vi "Run.vi"(8 "error in (no error)":errorcluster, 10 "OTP Cluster Out":T1, 11 "RF Powers in":refnum<class "RF Power.lvclass">) -> (0 "error out":errorcluster, 1 "Parameters":cluster{"Name":string, "Value":string}[](array[cluster]), 2 "Canceled":bool, 3 "RF Powers out":refnum<class "RF Power.lvclass">)   [LabVIEW 2020, in "RF Power.lvclass"]
doc: "This is the main test vi. It is here that the test is implemented."
uses:
  RF Power.lvclass
  Measurement.lvclass
  Devices/Device.lvclass
  Devices/Controls/Change setting mode enum.ctl
  Devices/PIC-device/PIC-Device.lvclass
  Support VI/Update parameters (single).vi
  Instruments/Power Supply/Power Supply.lvclass
  Support VI/Update parameters (array).vi
  Instruments/Digital Multimeter/Digital Multimeter.lvclass
  XML Handler/XML Handler.lvclass
  Path Control/Paths.ctl
  Path Control/PathControl.lvclass
  Instruments/Signal Generator/Signal Generator.lvclass
  Controls/Loop order.ctl
  Controls/Run states.ctl
  Instruments/Power Meter/Power Meter.lvclass
  C:/Sandbox/Git_Sandbox/WiSpry Test Framework source code (LV20)/WiSpry Test Framework/Measurements/Measurement.lvclass
  Controls/OTP_Cluster.ctl
panel:
  in  "Cancel Button":bool
  out "Power Meter reading (dBm)":dbl[](array[numeric])
  out "Estimated finish time":timestamp format="%<%X>T"
  out "Parameters":string
  out "Current Frequency [Hz]":dbl format="%#_6p"
  out "Current Power [dBm]":dbl
  out "XY Graph":cluster{dbl[], dbl[]}[](graph)
  out "Progress":u8(slide) scale=0.0..100.0
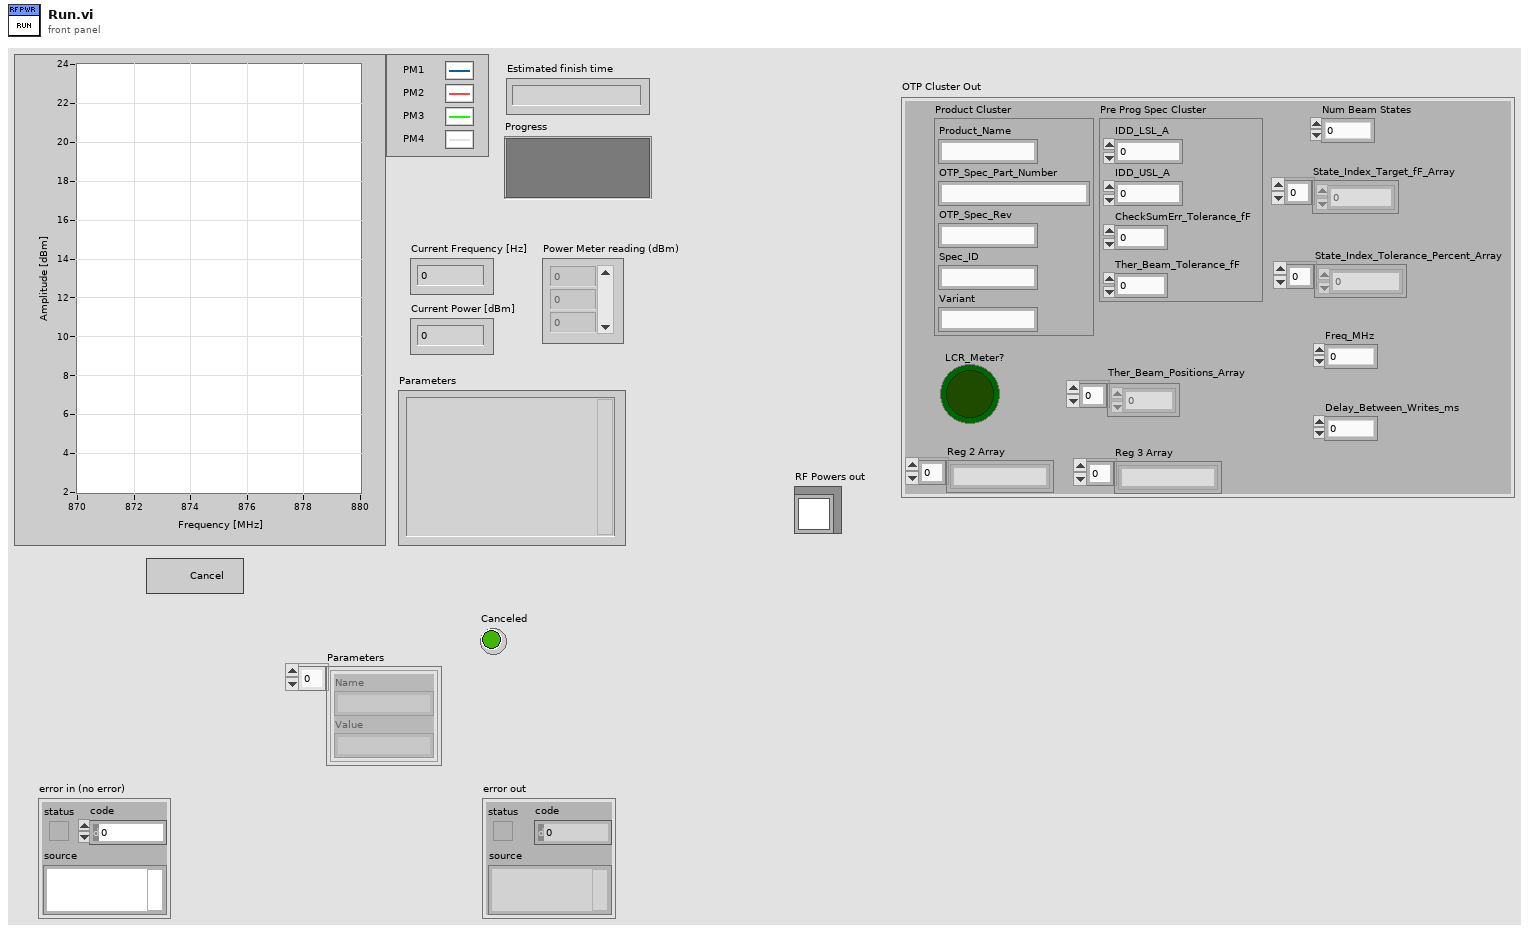
[diagram p1: front panel]
types:
  T1 = typedef "OTP_Cluster.ctl" = cluster{"Product Cluster":cluster{"Product_Name":string, "OTP_Spec_Part_Number":string, "OTP_Spec_Rev":string, "Spec_ID":string, "Variant":string}, "Pre Prog Spec Cluster":cluster{"IDD_LSL_A":dbl, "IDD_USL_A":dbl, "CheckSumErr_Tolerance_fF":dbl, "Ther_Beam_Tolerance_fF":dbl}, "LCR_Meter?":bool, "Reg 2 Array":string[], "Reg 3 Array":string[], "Num Beam States":i32, "State_Index_Target_fF_Array":dbl[], "State_Index_Tolerance_Percent_Array":dbl[], "Freq_MHz":dbl, "Delay_Between_Writes_ms":i32, "Ther_Beam_Positions_Array":i8[]}
  T2 = typedef "RF Power.lvclass/Run states.ctl" = enum16{"Init", "Set Device", "Set Power", "Set Frequency", "Read Environment", "Measure", "Done"}
  T3 = typedef "RF Power.lvclass/Loop order.ctl" = enum16{"Device -> Power -> Frequency", "Device -> Frequency -> Power"}
  T4 = enum32{"Invalid", "Standard", "Closed", "Hidden", "Minimized", "Maximized"}
  T5 = typedef "PIC-Device.lvclass/Change setting mode enum.ctl" = enum16{"Init", "Next", "Reset"}
  T6 = typedef "PathControl.lvclass/Paths.ctl" = enum16{"SigGen 1 -> DUT", "SigGen 2 -> DUT", "SigGen 1 -> PM 1", "SigGen 1 -> PM 2", "DUT -> SA", "DUT -> PM 2", "VSG -> DUT", "SigGen 2 -> PM 1", "SigGen 2 -> PM 2"}
  T7 = typedef "RF Power.lvclass/Config info.ctl" = cluster{"Frequency (MHz)":string, "Power (dBm)":string, "Loop order":T3, "SG loss":bool, "PM loss":bool, "SG":i32}
  T8 = typedef "XML Handler.lvclass/Result Cluster.ctl" = cluster{"Name":string, "Value":string}
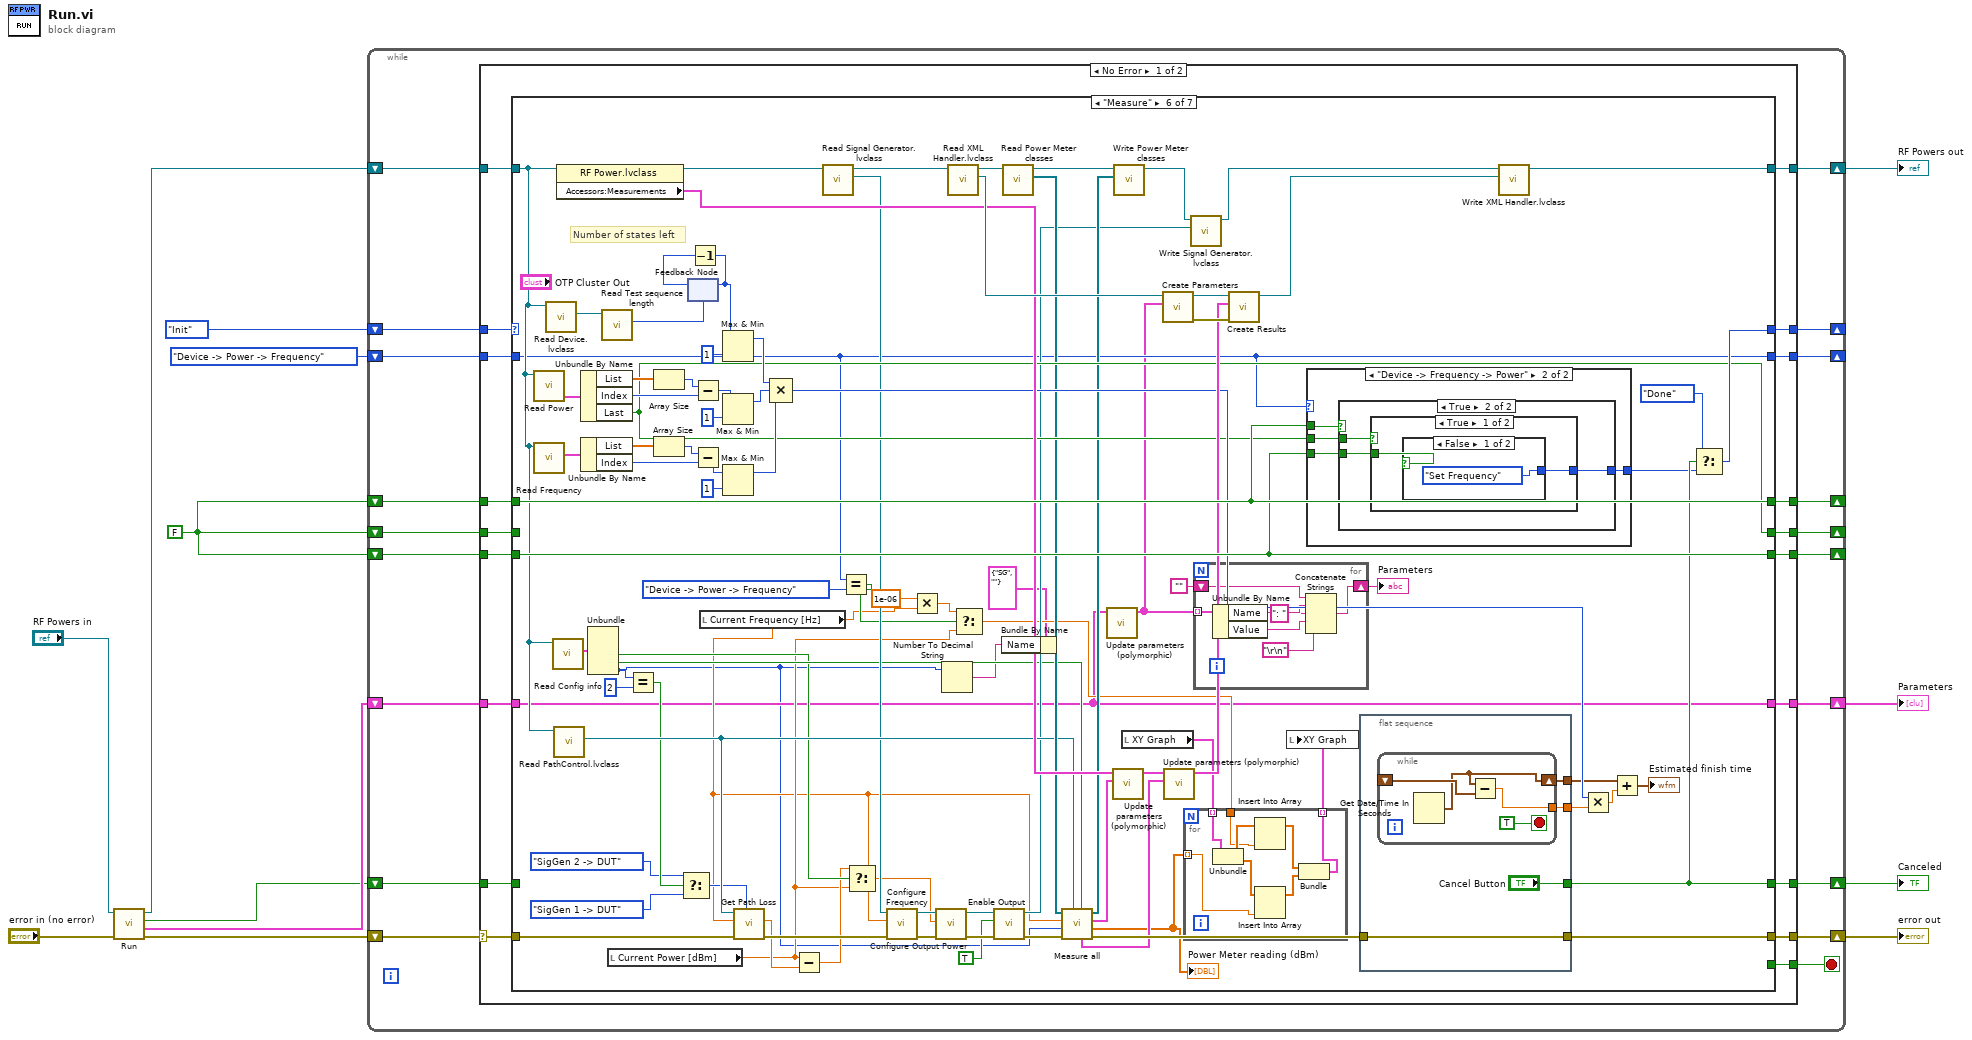
[diagram p0: block diagram]
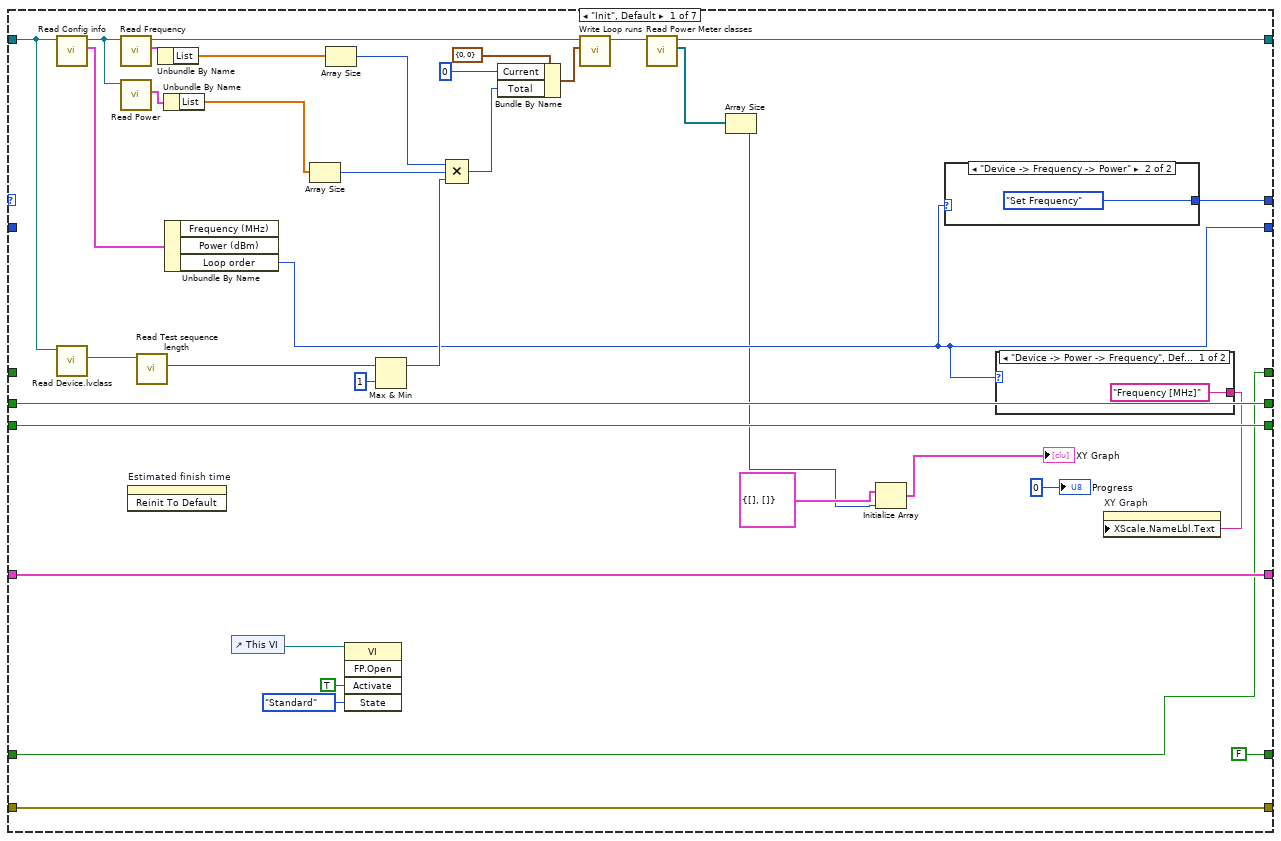
[diagram p2: hidden frame]
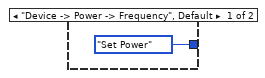
[diagram p3: hidden frame]
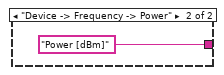
[diagram p4: hidden frame]
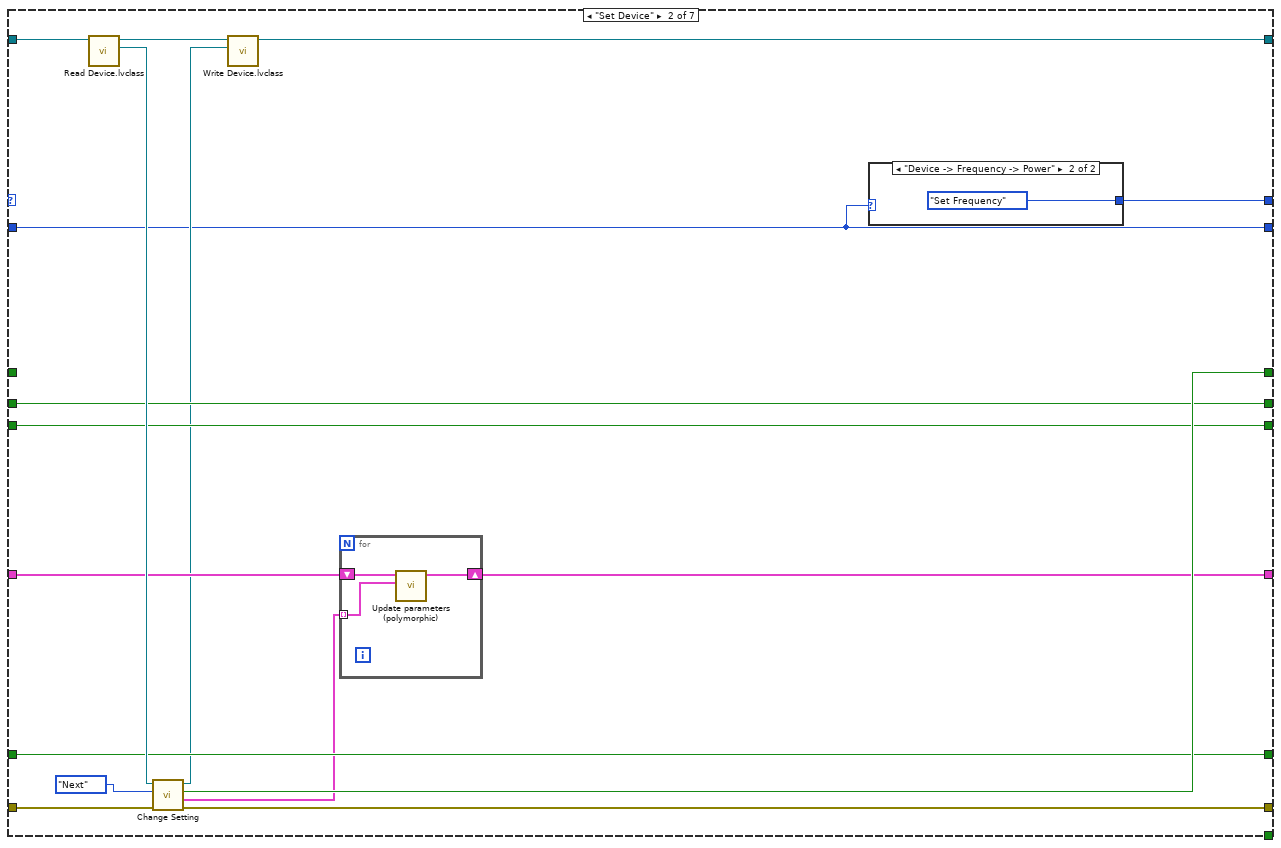
[diagram p5: hidden frame]
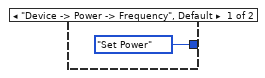
[diagram p6: hidden frame]
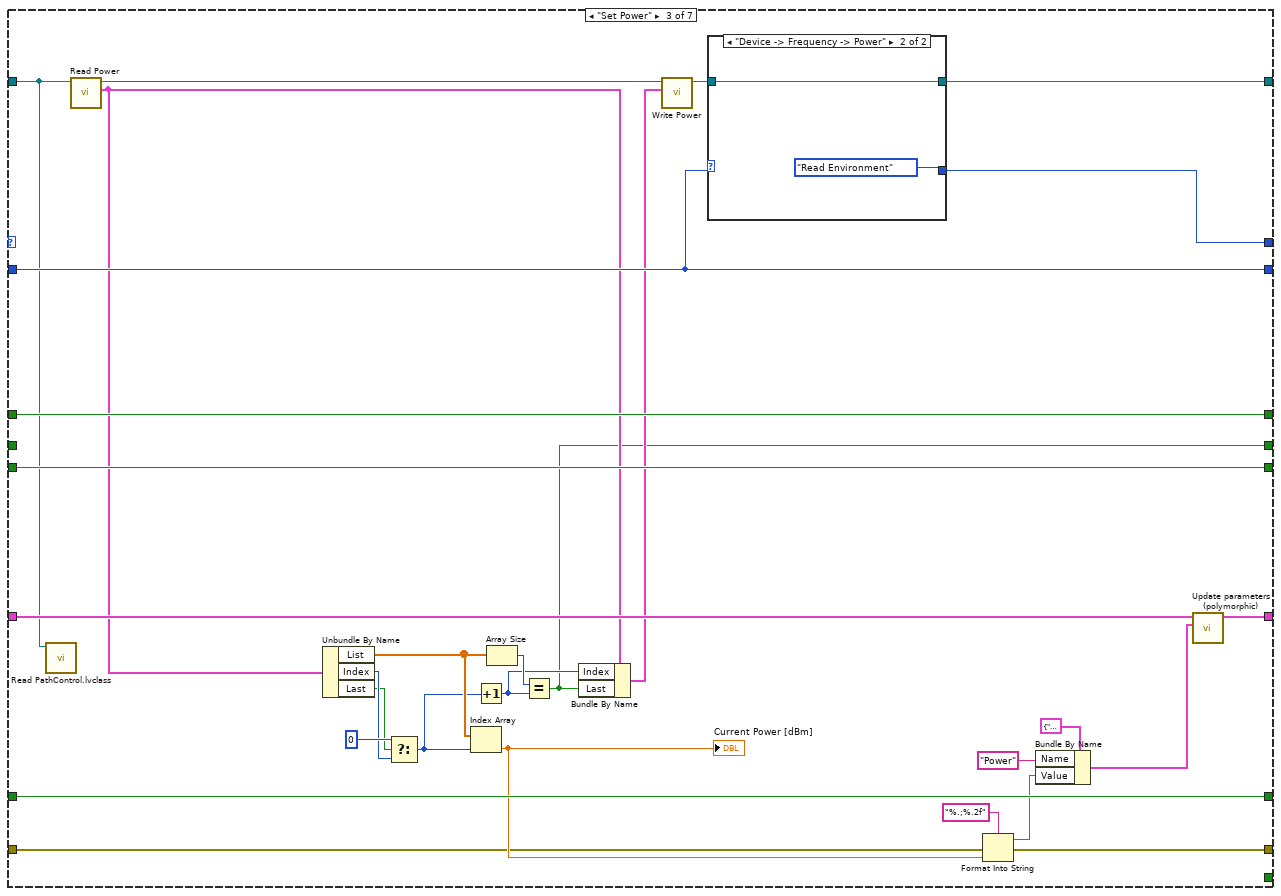
[diagram p7: hidden frame]
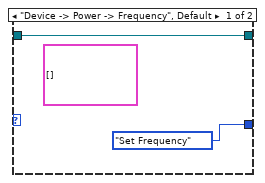
[diagram p8: hidden frame]
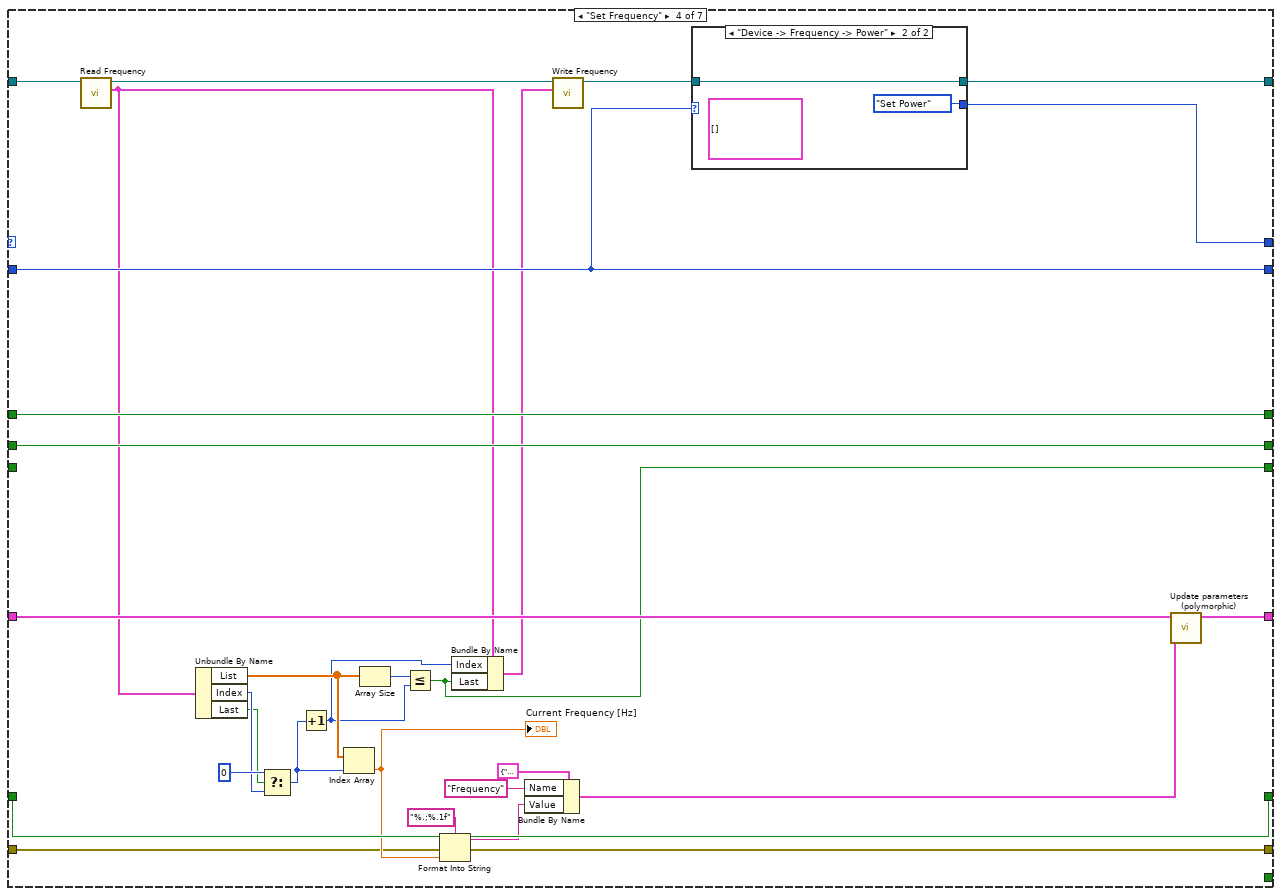
[diagram p9: hidden frame]
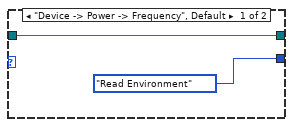
[diagram p10: hidden frame]
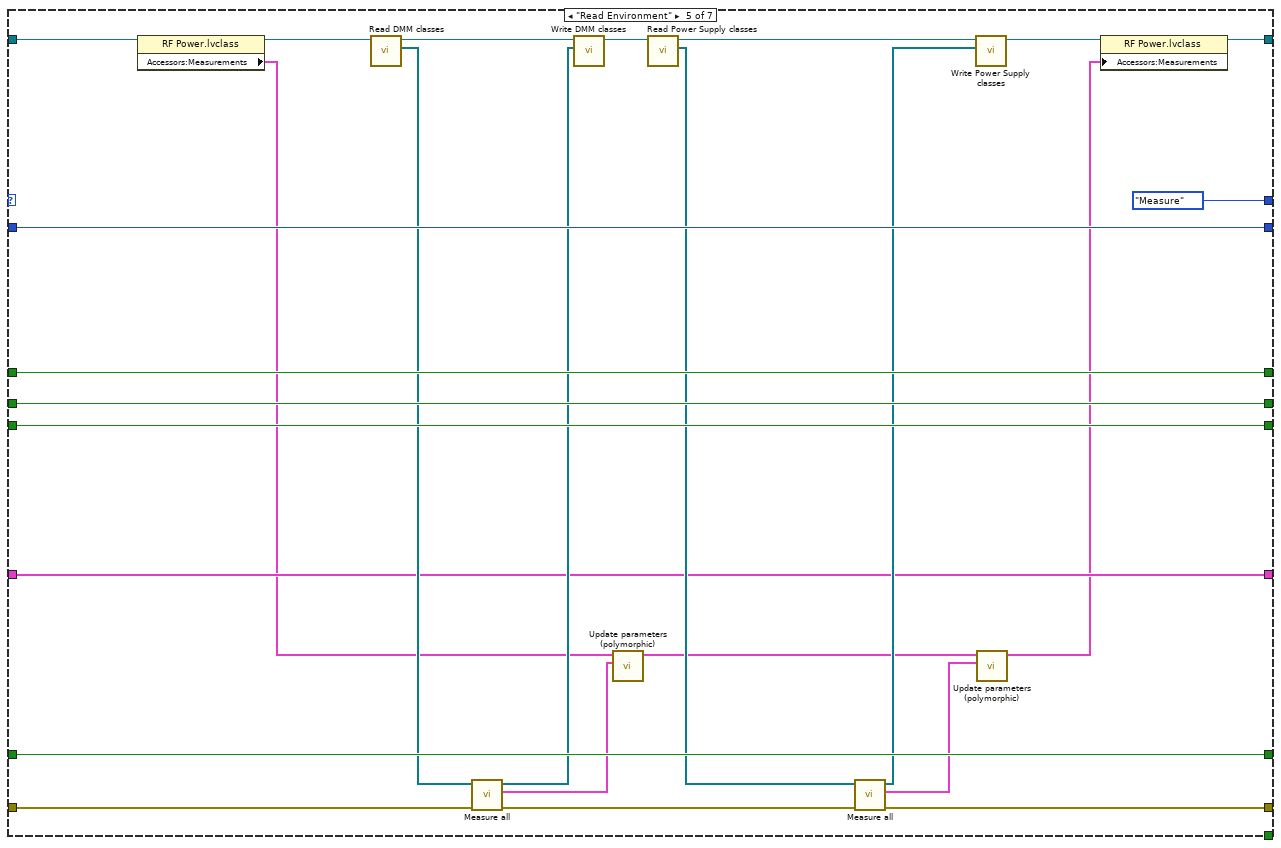
[diagram p11: hidden frame]
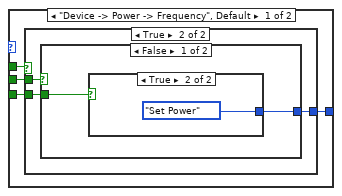
[diagram p12: hidden frame]
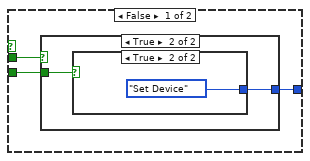
[diagram p13: hidden frame]
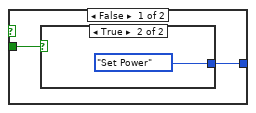
[diagram p14: hidden frame]
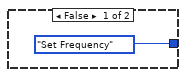
[diagram p15: hidden frame]
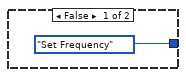
[diagram p16: hidden frame]
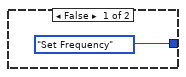
[diagram p17: hidden frame]
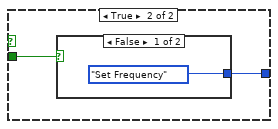
[diagram p18: hidden frame]
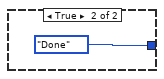
[diagram p19: hidden frame]
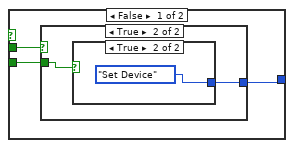
[diagram p20: hidden frame]
diagram:
  w11 = FALSE
  n1 = call-parent "Run.vi"("error in (no error)"="error in (no error)", "Measurements in"="RF Powers in") -> ("error out"=w6:errorcluster, "Parameters"=w5:cluster{"Name":string, "Value":string}[], "Canceled"=w4:bool, "Measurements out"=w7:refnum<class "RF Power.lvclass">)  [unwired: 5 in, 1 out]
  n2 = while {
    shift-right: [w30] -> w9
    shift-left: w6 -> [w16]
    shift-right: [w14] -> w1
    shift-left: w7 -> [w15]
    shift-right: [w27] -> _
    shift-left: Run_states."Init" ("Run states") -> [w32]
    shift-right: [w29] -> _
    shift-left: w11 -> [w28]
    shift-right: [w26] -> _
    shift-left: Loop_order."Device -> Power -> Frequency" ("Loop order") -> [w25]
    shift-right: [w22] -> _
    shift-left: w11 -> [w24]
    shift-right: [w21] -> _
    shift-left: w11 -> [w23]
    shift-right: [w20] -> w8
    shift-left: w4 -> [w19]
    shift-right: [w17] -> w10
    shift-left: w5 -> [w18]
    stop <- w31 stop-if-true
    n3 = case shown="No Error" w16 {
      selector: w16 -> [w50 w414]
      tunnel: w15 -> [w34 w415]
      tunnel: w32 -> [w51 _]
      tunnel: [w33 w415] -> w14
      tunnel: [w49 TRUE] -> w31
      tunnel: [w48 w414] -> w30
      tunnel: [w47 _] -> w29
      tunnel: w28 -> [w46 _]
      tunnel: [w45 _] -> w27
      tunnel: [w44 _] -> w26
      tunnel: w25 -> [w43 _]
      tunnel: w24 -> [w42 _]
      tunnel: w23 -> [w41 _]
      tunnel: [w40 _] -> w22
      tunnel: [w39 _] -> w21
      tunnel: [w38 _] -> w20
      tunnel: w19 -> [w37 _]
      tunnel: w18 -> [w36 w413]
      tunnel: [w35 w413] -> w17
      frame No Error {
        n4 = case shown="\"Measure\"" w51 {
          tunnel: w34 -> [w86 w109 w116 w155 w186 w249 w374]
          tunnel: [w55 w93 w138 w171 w187 w298 w374] -> w33
          tunnel: w50 -> [w69 w106 w115 w152 w191 w247 w399]
          tunnel: [_ _ _ _ _ _ TRUE] -> w49
          tunnel: [w69 w100 w118 w151 w190 w297 w397] -> w48
          tunnel: [w63 w105 w143 w176 w206 w296 w408] -> w47
          tunnel: w46 -> [_ _ w143 w176 w206 w296 w408]
          tunnel: [w65 w94 w141 w174 Run_states."Measure" ("Run states") w292 Run_states."Init" ("Run states")] -> w45
          tunnel: [w64 w95 w142 w175 w205 w221 w409] -> w44
          tunnel: w43 -> [_ w95 w142 w175 w205 w221 w409]
          tunnel: w42 -> [w82 w104 _ w173 w204 _ w407]
          tunnel: w41 -> [w81 w103 w140 _ w203 w295 w406]
          tunnel: [w82 w104 w117 w173 w204 w260 w407] -> w40
          tunnel: [w81 w103 w140 w148 w203 w295 w406] -> w39
          tunnel: [FALSE ("Last setting") w102 w139 w172 w202 w294 w403] -> w38
          tunnel: w37 -> [w63 w102 w139 w172 w202 _ w403]
          tunnel: w36 -> [w72 w99 w137 w170 w184 w211 w402]
          tunnel: [w72 w97 w136 w169 w184 w211 w402] -> w35
          frame "Init", Default {
            n5 = call-dynamic "Read Config info.vi"("RF Power in"=w86) -> ("Config info"=w87:T7, "RF Power out"=w88:refnum<class "RF Power.lvclass">)  [unwired: 9 in]
            n6 = call "Read Device.lvclass.vi"("Measurements in"=w86) -> ("Device.lvclass"=w83:refnum<class "Device.lvclass">)  [unwired: 9 in, 1 out]
            n7 = call-dynamic "Read Frequency.vi"("RF Power in"=w88) -> ("Frequency"=w80:cluster{"List":dbl[], "Index":i32, "Last":bool}, "RF Power out"=w77:refnum<class "RF Power.lvclass">)  [unwired: 9 in]
            n8 = call-dynamic "Read Power.vi"("RF Power in"=w88) -> ("Power"=w78:cluster{"List":dbl[], "Index":i32, "Last":bool})  [unwired: 9 in, 1 out]
            n9 = invoke on="Estimated finish time" class="AbsTime (strict)" method="Reinit To Default"() -> ()  [unwired: 3 in, 3 out]
            n10 = call-dynamic "Read Test sequence length.vi"("Device in"=w83) -> ("Test sequence length"=w68:i32)  [unwired: 8 in, 2 out]
            n11 = Unbundle By Name(w80) -> ("List"=w79:dbl[])
            n12 = Unbundle By Name(w78) -> ("List"=w61:dbl[])
            n13 = Unbundle By Name(w87) -> ("Loop order"=w64:T3)  [unwired: 2 out]
            n14 = control-ref of="This VI"() -> (w60:refnum<vi>)
            n15 = Array Size(array=w61) -> (size(s)=w84:i32)
            n16 = Array Size(array=w79) -> (size(s)=w85:i32)
            n17 = invoke class="VI" method="FP.Open"(reference=w60, "Activate"=TRUE ("Activate?"), "State"=T4."Standard") -> ()  [unwired: 2 in, 5 out]
            n18 = Max & Min(x=w68, y=1) -> (max(x,y)=w67:i32)  [unwired: 1 out]
            n19 = Compound Arithmetic op=MULTIPLY(w85, w84, w67) -> (w73:i32)
            n20 = Bundle By Name(cluster=cluster{"Current":u32, "Total":u32} {"Current"=0, "Total"=0} ("Loop runs"), "Current"=u32 0, "Total"=w73) -> (w74:cluster{"Current":u32, "Total":u32})
            n21 = call "Write Loop runs.vi"("Loop runs"=w74, "Measurements in"=w77) -> ("Measurements out"=w56:refnum<class "RF Power.lvclass">)  [unwired: 9 in]
            n22 = call-dynamic "Read Power Meter classes.vi"("RF Power in"=w56) -> ("Power Meter classes"=w54:refnum<class "Power Meter.lvclass">[], "RF Power out"=w55:refnum<class "RF Power.lvclass">)  [unwired: 9 in]
            n23 = Array Size(array=w54) -> (size(s)=w53:i32)
            n24 = Initialize Array(cluster{dbl[], dbl[]} {[], []}, w53) -> (→"XY Graph":cluster{dbl[], dbl[]}[])
            n25 = case shown="\"Device -> Frequency -> Power\"" w64 {
              tunnel: [Run_states."Set Power" ("Run states") Run_states."Set Frequency" ("Run states")] -> w65
              frame "Device -> Power -> Frequency", Default {
              }
              frame "Device -> Frequency -> Power" {
              }
            }
            n26 = case shown="\"Device -> Power -> Frequency\", Default" w64 {
              tunnel: ["Frequency [MHz]" "Power [dBm]"] -> w70
              frame "Device -> Power -> Frequency", Default {
              }
              frame "Device -> Frequency -> Power" {
              }
            }
            n27 = property on="XY Graph" class="XYGraph (strict)"("XScale.NameLbl.Text"=w70) -> ()  [unwired: 2 in, 2 out]
            "Progress" <- u8 0 ("Progress")
          }
          frame "Set Device" {
            n28 = call "Read Device.lvclass.vi"("Measurements in"=w109) -> ("Device.lvclass"=w108:refnum<class "Device.lvclass">, "Measurements out"=w101:refnum<class "RF Power.lvclass">)  [unwired: 9 in]
            n29 = call-dynamic "Change Setting.vi"("error in (no error)"=w106, "Change setting mode"=Change_setting_mode_enum."Next", "Device in"=w108) -> ("error out"=w100:errorcluster, "Changes"=w98:cluster{"Name":string, "Value":string}[], "Last setting"=w105:bool, "Device out"=w96:refnum<class "Device.lvclass">)  [unwired: 5 in]
            n30 = call "Write Device.lvclass.vi"("Device.lvclass"=w96, "Measurements in"=w101) -> ("Measurements out"=w93:refnum<class "RF Power.lvclass">)  [unwired: 9 in]
            n31 = for {
              shift-right: [w113] -> w97
              shift-left: w99 -> [w114]
              tunnel: w98 -> [w112] mode=indexing
              n32 = call-poly "Update parameters (polymorphic).vi"("New Parameter"=w112, "Parameters"=w114) -> ("Parameters Out"=w113:cluster{"Name":string, "Value":string}[])  [unwired: 9 in]
            }
            n33 = case shown="\"Device -> Frequency -> Power\"" w95 {
              tunnel: [Run_states."Set Power" ("Run states") Run_states."Set Frequency" ("Run states")] -> w94
              frame "Device -> Power -> Frequency", Default {
              }
              frame "Device -> Frequency -> Power" {
              }
            }
          }
          frame "Set Power" {
            n34 = call "Read PathControl.lvclass.vi"("Measurements in"=w116) -> ()  [unwired: 9 in, 2 out]
            n35 = call-dynamic "Read Power.vi"("RF Power in"=w116) -> ("Power"=w134:cluster{"List":dbl[], "Index":i32, "Last":bool}, "RF Power out"=w135:refnum<class "RF Power.lvclass">)  [unwired: 9 in]
            n36 = Unbundle By Name(w134) -> ("List"=w121:dbl[], "Index"=w132:i32, "Last"=w130:bool)
            n37 = Select(t=0, s=w130, f=w132) -> (s? t:f=w120:i32)
            n38 = Index Array(array=w121, index=w120) -> (element=w119:dbl)
            "Current Power [dBm]" <- w119
            n39 = Increment(x=w120) -> (x+1=w128:i32)
            n40 = Array Size(array=w121) -> (size(s)=w129:i32)
            n41 = Equal?(x=w129, y=w128) -> (x = y?=w117:bool)
            n42 = Bundle By Name(cluster=w134, "Index"=w128, "Last"=w117) -> (w131:cluster{"List":dbl[], "Index":i32, "Last":bool})
            n43 = call-dynamic "Write Power.vi"("Power"=w131, "RF Power in"=w135) -> ("RF Power out"=w122:refnum<class "RF Power.lvclass">)  [unwired: 9 in]
            n44 = case shown="\"Device -> Frequency -> Power\"" w142 {
              tunnel: [Run_states."Set Frequency" ("Run states") Run_states."Read Environment" ("Run states")] -> w141
              tunnel: w122 -> [w144 w147]
              tunnel: [w144 w147] -> w138
              frame "Device -> Power -> Frequency", Default {
                (unwired) cluster{"Array":dbl[], "Array":dbl[]}[] [] ("Graph Data")
              }
              frame "Device -> Frequency -> Power" {
              }
            }
            n45 = Format Into String(format string="%.;%.2f", error in=w115, w119) -> (resulting string=w124:string, error out=w118:errorcluster)  [unwired: 1 in]
            n46 = Bundle By Name(cluster=cluster{"Name":string, "Value":string} {"Name"="", "Value"=""} ("Change"), "Name"="Power", "Value"=w124) -> (w123:cluster{"Name":string, "Value":string})
            n47 = call-poly "Update parameters (polymorphic).vi"("New Parameter"=w123, "Parameters"=w137) -> ("Parameters Out"=w136:cluster{"Name":string, "Value":string}[])  [unwired: 9 in]
          }
          frame "Set Frequency" {
            n48 = call-dynamic "Read Frequency.vi"("RF Power in"=w155) -> ("Frequency"=w149:cluster{"List":dbl[], "Index":i32, "Last":bool}, "RF Power out"=w154:refnum<class "RF Power.lvclass">)  [unwired: 9 in]
            n49 = Unbundle By Name(w149) -> ("List"=w165:dbl[], "Index"=w167:i32, "Last"=w166:bool)
            n50 = Select(t=0, s=w166, f=w167) -> (s? t:f=w163:i32)
            n51 = Increment(x=w163) -> (x+1=w162:i32)
            n52 = Index Array(array=w165, index=w163) -> (element=w157:dbl)
            "Current Frequency [Hz]" <- w157
            n53 = Array Size(array=w165) -> (size(s)=w164:i32)
            n54 = Less Or Equal?(x=w164, y=w162) -> (x <= y?=w148:bool)
            n55 = Format Into String(format string="%.;%.1f", error in=w152, w157) -> (resulting string=w158:string, error out=w151:errorcluster)  [unwired: 1 in]
            n56 = Bundle By Name(cluster=w149, "Index"=w162, "Last"=w148) -> (w150:cluster{"List":dbl[], "Index":i32, "Last":bool})
            n57 = Bundle By Name(cluster=cluster{"Name":string, "Value":string} {"Name"="", "Value"=""} ("Change"), "Name"="Frequency", "Value"=w158) -> (w156:cluster{"Name":string, "Value":string})
            n58 = call-dynamic "Write Frequency.vi"("Frequency"=w150, "RF Power in"=w154) -> ("RF Power out"=w153:refnum<class "RF Power.lvclass">)  [unwired: 9 in]
            n59 = case shown="\"Device -> Frequency -> Power\"" w175 {
              tunnel: [Run_states."Read Environment" ("Run states") Run_states."Set Power" ("Run states")] -> w174
              tunnel: [w178 w180] -> w171
              tunnel: w153 -> [w178 w180]
              frame "Device -> Power -> Frequency", Default {
              }
              frame "Device -> Frequency -> Power" {
                (unwired) cluster{"Array":dbl[], "Array":dbl[]}[] [] ("Graph Data")
              }
            }
            n60 = call-poly "Update parameters (polymorphic).vi"("New Parameter"=w156, "Parameters"=w170) -> ("Parameters Out"=w169:cluster{"Name":string, "Value":string}[])  [unwired: 9 in]
          }
          frame "Read Environment" {
            n61 = property class="RF Power.lvclass"(reference=w186) -> (reference out=w185:refnum<class "RF Power.lvclass">, "Accessors:Measurements"=w183:cluster{"Name":string, "Value":string}[])  [unwired: 1 in, 1 out]
            n62 = call-dynamic "Read DMM classes.vi"("Measurements in"=w185) -> ("DMM classes"=w196:refnum<class "Digital Multimeter.lvclass">[], "Measurements out"=w201:refnum<class "RF Power.lvclass">)  [unwired: 9 in]
            n63 = call "Measure all.vi"("error in (no error)"=w191, "Digital Multimeters in"=w196) -> ("error out"=w194:errorcluster, "Measurements"=w193:T8[], "Digital Multimeters out"=w195:refnum<class "Digital Multimeter.lvclass">[])  [unwired: 5 in, 2 out]
            n64 = call-dynamic "Write DMM classes.vi"("DMM classes"=w195, "Measurements in"=w201) -> ("Measurements out"=w198:refnum<class "RF Power.lvclass">)  [unwired: 9 in]
            n65 = call-poly "Update parameters (polymorphic).vi"("New Parameters"=w193, "Parameters"=w183) -> ("Parameters Out"=w192:cluster{"Name":string, "Value":string}[])  [unwired: 9 in]
            n66 = call-dynamic "Read Power Supply classes.vi"("Measurements in"=w198) -> ("Power Supply classes"=w200:refnum<class "Power Supply.lvclass">[], "Measurements out"=w189:refnum<class "RF Power.lvclass">)  [unwired: 9 in]
            n67 = call "Measure all.vi"("error in (no error)"=w194, "Power Supplies in"=w200) -> ("error out"=w190:errorcluster, "Measurements"=w197:T8[], "Power Supplies out"=w199:refnum<class "Power Supply.lvclass">[])  [unwired: 5 in, 2 out]
            n68 = call-dynamic "Write Power Supply classes.vi"("Power Supply classes"=w199, "Measurements in"=w189) -> ("Measurements out"=w188:refnum<class "RF Power.lvclass">)  [unwired: 9 in]
            n69 = call-poly "Update parameters (polymorphic).vi"("New Parameters"=w197, "Parameters"=w192) -> ("Parameters Out"=w182:cluster{"Name":string, "Value":string}[])  [unwired: 9 in]
            n70 = property class="RF Power.lvclass"(reference=w188, "Accessors:Measurements"=w182) -> (reference out=w187:refnum<class "RF Power.lvclass">)  [unwired: 1 in, 1 out]
          }
          frame "Measure" {
            # "Number of states left"
            n71 = call-dynamic "Read Power.vi"("RF Power in"=w249) -> ("Power"=w282:cluster{"List":dbl[], "Index":i32, "Last":bool})  [unwired: 9 in, 1 out]
            n72 = call-dynamic "Read Frequency.vi"("RF Power in"=w249) -> ("Frequency"=w281:cluster{"List":dbl[], "Index":i32, "Last":bool})  [unwired: 9 in, 1 out]
            n73 = call "Read Device.lvclass.vi"("Measurements in"=w249) -> ("Device.lvclass"=w285:refnum<class "Device.lvclass">)  [unwired: 9 in, 1 out]
            n74 = call-dynamic "Read Config info.vi"("RF Power in"=w249) -> ("Config info"=w250:T7)  [unwired: 9 in, 1 out]
            n75 = call "Read PathControl.lvclass.vi"("Measurements in"=w249) -> ("PathControl.lvclass"=w248:refnum<class "PathControl.lvclass">)  [unwired: 9 in, 1 out]
            n76 = property class="RF Power.lvclass"(reference=w249) -> (reference out=w226:refnum<class "RF Power.lvclass">, "Accessors:Measurements"=w288:cluster{"Name":string, "Value":string}[])  [unwired: 1 in, 1 out]
            n77 = Unbundle By Name(w282) -> ("List"=w280:dbl[], "Index"=w278:i32, "Last"=w260:bool)
            n78 = Unbundle By Name(w281) -> ("List"=w251:dbl[], "Index"=w224:i32)
            n79 = Unbundle(w250) -> ("SG loss"=w229:bool, "PM loss"=w235:bool, "SG"=w207:i32)  [unwired: 3 out]
            n80 = call-dynamic "Read Test sequence length.vi"("Device in"=w285) -> ("Test sequence length"=w283:i32)  [unwired: 8 in, 2 out]
            n81 = local read "Current Power [dBm]"() -> (w218:dbl)
            n82 = Equal?(x=w207, y=2) -> (x = y?=w233:bool)
            n83 = Array Size(array=w280) -> (size(s)=w279:i32)
            n84 = Array Size(array=w251) -> (size(s)=w270:i32)
            n85 = Select(t=Paths."SigGen 2 -> DUT" ("Path"), s=w233, f=Paths."SigGen 1 -> DUT" ("Path")) -> (s? t:f=w230:T6)
            n86 = feedback #1(w283) -> (w284:i32)
            n87 = Decrement(x=w284) -> (x-1=w268:i32)
            n88 = feedback-in #1(w268) -> ()
            n89 = Subtract(x=w279, y=w278) -> (x-y=w265:i32)
            n90 = Subtract(x=w270, y=w224) -> (x-y=w269:i32)
            n91 = local read "Current Frequency [Hz]"() -> (w214:dbl)
            n92 = Max & Min(x=w268, y=1) -> (max(x,y)=w266:i32)  [unwired: 1 out]
            n93 = Max & Min(x=w265, y=1) -> (max(x,y)=w264:i32)  [unwired: 1 out]
            n94 = Max & Min(x=w269, y=1) -> (max(x,y)=w263:i32)  [unwired: 1 out]
            n95 = call "Get Path Loss.vi"("Path"=w230, "error in (no error)"=w247, "Frequency [Hz]"=w214, "PathControl in"=w248) -> ("error out"=w242:errorcluster, "Insertion Loss (dB)"=w236:dbl)  [unwired: 4 in, 2 out]
            n96 = Compound Arithmetic op=MULTIPLY(w266, w264, w263) -> (w277:i32)
            n97 = Subtract(x=w218, y=w236) -> (x-y=w228:dbl)
            n98 = call-dynamic "Read Signal Generator.lvclass.vi"("RF Power in"=w226) -> ("Signal Generator.lvclass"=w241:refnum<class "Signal Generator.lvclass">, "RF Power out"=w225:refnum<class "RF Power.lvclass">)  [unwired: 9 in]
            n99 = Equal?(x=w221, y=Loop_order."Device -> Power -> Frequency") -> (x = y?=w219:bool)
            n100 = Select(t=w228, s=w229, f=w218) -> (s? t:f=w227:dbl)
            n101 = call-dynamic "Configure Frequency.vi"("error in (no error)"=w242, "Frequency [Hz]"=w214, "Signal Generator in"=w241) -> ("error out"=w245:errorcluster, "Signal Generator out"=w246:refnum<class "Signal Generator.lvclass">)  [unwired: 7 in]
            n102 = Multiply(x=1e-06, y=w214) -> (x*y=w213:dbl)
            n103 = call-dynamic "Configure Output Power.vi"("error in (no error)"=w245, "Output Power [dBm]"=w227, "Signal Generator in"=w246) -> ("error out"=w243:errorcluster, "Signal Generator out"=w244:refnum<class "Signal Generator.lvclass">)  [unwired: 7 in]
            n104 = Number To Decimal String(number=w207) -> (decimal integer string=w208:string)  [unwired: 1 in]
            n105 = call "Read XML Handler.lvclass.vi"("Measurements in"=w225) -> ("XML Handler.lvclass"=w291:refnum<class "XML Handler.lvclass">, "Measurements out"=w253:refnum<class "RF Power.lvclass">)  [unwired: 9 in]
            n106 = Select(t=w213, s=w219, f=w218) -> (s? t:f=w217:dbl)
            n107 = call-dynamic "Enable Output.vi"("error in (no error)"=w243, "Output Enable (F)"=TRUE, "Signal Generator in"=w244) -> ("error out"=w239:errorcluster, "Signal Generator out"=w240:refnum<class "Signal Generator.lvclass">)  [unwired: 7 in]
            n108 = Bundle By Name(cluster=cluster{"Name":string, "Value":string} {"Name"="SG", "Value"=""} ("New Parameter"), "Name"=w208) -> ()  [unwired: 1 out]
            n109 = call-dynamic "Read Power Meter classes.vi"("RF Power in"=w253) -> ("Power Meter classes"=w255:refnum<class "Power Meter.lvclass">[], "RF Power out"=w254:refnum<class "RF Power.lvclass">)  [unwired: 9 in]
            n110 = call "Measure all.vi"("Path loss compensation"=w235, "PathControl in"=w248, "Error In"=w239, "SG"=w207, "Frequency"=w214, "Power Meter classes"=w255) -> ("Error Out"=w258:errorcluster, "Power readings"=w222:dbl[], "Power results"=w257:T8[], "Power Meter classes"=w256:refnum<class "Power Meter.lvclass">[], "Calibration values"=w252:cluster{"Name":string, "Value":string}[])  [unwired: 1 in]
            "Power Meter reading (dBm)" <- w222
            n111 = call-poly "Update parameters (polymorphic).vi"("Parameters"=w211) -> ("Parameters Out"=w210:cluster{"Name":string, "Value":string}[])  [unwired: 10 in]
            n112 = call-poly "Update parameters (polymorphic).vi"("New Parameters"=w257, "Parameters"=w288) -> ("Parameters Out"=w287:cluster{"Name":string, "Value":string}[])  [unwired: 9 in]
            n113 = call-dynamic "Write Power Meter classes.vi"("Power Meter classes"=w256, "RF Power in"=w254) -> ("RF Power out"=w238:refnum<class "RF Power.lvclass">)  [unwired: 9 in]
            n114 = local read "XY Graph"() -> (w216:cluster{dbl[], dbl[]}[])
            n115 = call "Create Parameters.vi"("Parameters"=w210, "XML Handler in"=w291) -> ("error out"=w289:errorcluster, "XML Handler out"=w290:refnum<class "XML Handler.lvclass">)  [unwired: 8 in]
            n116 = call-poly "Update parameters (polymorphic).vi"("New Parameters"=w252, "Parameters"=w287) -> ("Parameters Out"=w286:cluster{"Name":string, "Value":string}[])  [unwired: 9 in]
            n117 = for {
              tunnel: w222 -> [w304] mode=indexing
              tunnel: w217 -> [w303]
              tunnel: w216 -> [w307] mode=indexing
              tunnel: [w300] -> w215 mode=indexing
              n118 = Unbundle(w307) -> (w306:dbl[], w305:dbl[])
              n119 = Insert Into Array(array=w306, new element=w303) -> (w302:dbl[])  [unwired: 1 in]
              n120 = Insert Into Array(array=w305, new element=w304) -> (w301:dbl[])  [unwired: 1 in]
              n121 = Bundle(w302, w301) -> (w300:cluster{dbl[], dbl[]})  [unwired: 1 in]
            }
            n122 = call-dynamic "Write Signal Generator.lvclass.vi"("Signal Generator.lvclass"=w240, "RF Power in"=w238) -> ("RF Power out"=w237:refnum<class "RF Power.lvclass">)  [unwired: 9 in]
            n123 = for {
              tunnel: w210 -> [w314] mode=indexing
              shift-right: [w308] -> w262
              shift-left: "" -> [w313]
              n124 = Unbundle By Name(w314) -> ("Name"=w312:string, "Value"=w310:string)
              n125 = Concatenate Strings(w313, w312, ": " ("string"), w310, "\r\n") -> (w308:string)
            }
            "Parameters" <- w262
            n126 = call "Create Results.vi"("error in (no error)"=w289, "Results"=w286, "XML Handler in"=w290) -> ("XML Handler out"=w299:refnum<class "XML Handler.lvclass">)  [unwired: 7 in, 1 out]
            n127 = local write "XY Graph"(w215) -> ()
            n128 = case shown="\"Device -> Frequency -> Power\"" w221 {
              tunnel: w296 -> [w318 w344]
              tunnel: w260 -> [w317 w343]
              tunnel: w295 -> [w316 w342]
              tunnel: [w315 w341] -> w293
              frame "Device -> Power -> Frequency", Default {
                n129 = case shown="True" w318 {
                  tunnel: w317 -> [w321 w332]
                  tunnel: w316 -> [w320 w331]
                  tunnel: [w319 w330] -> w315
                  frame False {
                    n130 = case shown="True" w321 {
                      tunnel: w320 -> [w323 w326]
                      tunnel: [w322 w327] -> w319
                      frame False {
                        n131 = case shown="True" w323 {
                          tunnel: [Run_states."Set Frequency" ("Run states") Run_states."Set Power" ("Run states")] -> w322
                          frame False {
                          }
                          frame True {
                          }
                        }
                      }
                      frame True {
                        n132 = case shown="True" w326 {
                          tunnel: [Run_states."Set Frequency" ("Run states") Run_states."Set Device" ("Run states")] -> w327
                          frame False {
                          }
                          frame True {
                          }
                        }
                      }
                    }
                  }
                  frame True {
                    n133 = case shown="False" w332 {
                      tunnel: w331 -> [w333 w337]
                      tunnel: [w334 w338] -> w330
                      frame False {
                        n134 = case shown="True" w333 {
                          tunnel: [Run_states."Set Frequency" ("Run states") Run_states."Set Power" ("Run states")] -> w334
                          frame False {
                          }
                          frame True {
                          }
                        }
                      }
                      frame True {
                        n135 = case shown="False" w337 {
                          tunnel: [Run_states."Set Frequency" ("Run states") Run_states."Done" ("Run states")] -> w338
                          frame False {
                          }
                          frame True {
                          }
                        }
                      }
                    }
                  }
                }
              }
              frame "Device -> Frequency -> Power" {
                n136 = case shown="True" w344 {
                  tunnel: w343 -> [w347 w355]
                  tunnel: w342 -> [w346 w354]
                  tunnel: [w345 w353] -> w341
                  frame False {
                    n137 = case shown="True" w347 {
                      tunnel: w346 -> [_ w350]
                      tunnel: [Run_states."Set Power" ("Run states") w349] -> w345
                      frame False {
                      }
                      frame True {
                        n138 = case shown="True" w350 {
                          tunnel: [Run_states."Set Frequency" ("Run states") Run_states."Set Device" ("Run states")] -> w349
                          frame False {
                          }
                          frame True {
                          }
                        }
                      }
                    }
                  }
                  frame True {
                    n139 = case shown="True" w355 {
                      tunnel: w354 -> [w357 _]
                      tunnel: [w356 Run_states."Set Power" ("Run states")] -> w353
                      frame True {
                        n140 = case shown="False" w357 {
                          tunnel: [Run_states."Set Frequency" ("Run states") Run_states."Done" ("Run states")] -> w356
                          frame False {
                          }
                          frame True {
                          }
                        }
                      }
                      frame False {
                      }
                    }
                  }
                }
              }
            }
            n141 = flat-sequence {
              tunnel: w258 -> [w364]
              tunnel: [w364] -> w297
              tunnel: ["Cancel Button"] -> w294
              tunnel: [w362] -> w276
              tunnel: [w361] -> w275
              frame #0 {
                n142 = while {
                  shift-right: [w365] -> w361
                  shift-left: _ -> [w366]
                  tunnel: [w367] -> w362
                  stop <- TRUE stop-if-true
                  n143 = Get Date/Time In Seconds() -> (seconds since 1Jan1904=w365:timestamp)
                  n144 = Subtract(x=w365, y=w366) -> (x-y=w367:dbl)
                }
              }
            }
            n145 = call "Write XML Handler.lvclass.vi"("XML Handler.lvclass"=w299, "Measurements in"=w237) -> ("Measurements out"=w298:refnum<class "RF Power.lvclass">)  [unwired: 9 in]
            n146 = Multiply(x=w277, y=w276) -> (x*y=w274:dbl)
            n147 = Add(x=w275, y=w274) -> (x+y=→"Estimated finish time":timestamp)
            n148 = Select(t=Run_states."Done" ("Run states"), s=w294, f=w293) -> (s? t:f=w292:T2)
          }
          frame "Done" {
            n149 = call "Read PathControl.lvclass.vi"("Measurements in"=w374) -> ("PathControl.lvclass"=w384:refnum<class "PathControl.lvclass">)  [unwired: 9 in, 1 out]
            n150 = call-dynamic "Read Frequency.vi"("RF Power in"=w374) -> ("Frequency"=w388:cluster{"List":dbl[], "Index":i32, "Last":bool})  [unwired: 9 in, 1 out]
            n151 = call-dynamic "Read Config info.vi"("RF Power in"=w374) -> ("Config info"=w381:T7)  [unwired: 9 in, 1 out]
            n152 = call-dynamic "Read Signal Generator.lvclass.vi"("RF Power in"=w374) -> ("Signal Generator.lvclass"=w395:refnum<class "Signal Generator.lvclass">)  [unwired: 9 in, 1 out]
            n153 = call-dynamic "Read Power.vi"("RF Power in"=w374) -> ("Power"=w392:cluster{"List":dbl[], "Index":i32, "Last":bool})  [unwired: 9 in, 1 out]
            n154 = Unbundle By Name(w388) -> ("List"=w387:dbl[], "Index"=w386:i32)
            n155 = Unbundle(w381) -> ("SG loss"=w373:bool, "SG"=w380:i32)  [unwired: 4 out]
            n156 = Unbundle By Name(w392) -> ("List"=w391:dbl[])
            n157 = Equal?(x=w380, y=2) -> (x = y?=w378:bool)
            n158 = Decrement(x=w386) -> (x-1=w385:i32)
            n159 = Select(t=Paths."SigGen 2 -> DUT" ("Path"), s=w378, f=Paths."SigGen 1 -> DUT" ("Path")) -> (s? t:f=w375:T6)
            n160 = Index Array(array=w387, index=w385) -> (element=w383:dbl)
            n161 = Array Max & Min(array=w391) -> (min value=w371:dbl)  [unwired: 3 out]
            n162 = control-ref of="This VI"() -> (w369:refnum<vi>)
            n163 = call "Get Path Loss.vi"("Path"=w375, "Frequency [Hz]"=w383, "PathControl in"=w384) -> ("Insertion Loss (dB)"=w382:dbl)  [unwired: 5 in, 3 out]
            n164 = Subtract(x=w371, y=w382) -> (x-y=w372:dbl)
            n165 = invoke class="VI" method="FP.Close"(reference=w369) -> ()  [unwired: 2 in, 3 out]
            n166 = Select(t=w372, s=w373, f=w371) -> (s? t:f=w370:dbl)
            n167 = call-dynamic "Configure Output Power.vi"("Output Power [dBm]"=w370, "Signal Generator in"=w395) -> ("error out"=w393:errorcluster, "Signal Generator out"=w394:refnum<class "Signal Generator.lvclass">)  [unwired: 8 in]
            n168 = call-dynamic "Read Power Meter classes.vi"("RF Power in"=w374) -> ("Power Meter classes"=w390:refnum<class "Power Meter.lvclass">[])  [unwired: 9 in, 1 out]
            n169 = call-dynamic "Enable Output.vi"("error in (no error)"=w393, "Output Enable (F)"=FALSE, "Signal Generator in"=w394) -> ("error out"=w400:errorcluster, "Signal Generator out"=w401:refnum<class "Signal Generator.lvclass">)  [unwired: 7 in]
            n170 = for {
              tunnel: w390 -> [w411] mode=indexing
              tunnel: [w410] -> w396 mode=indexing
              n171 = call-dynamic "Close Instrument.vi"("Instrument in"=w411) -> ("error out"=w410:errorcluster)  [unwired: 9 in, 1 out]
            }
            n172 = call-dynamic "Close Instrument.vi"("error in (no error)"=w400, "Instrument in"=w401) -> ("error out"=w398:errorcluster)  [unwired: 8 in, 1 out]
            n173 = Merge Errors(w399, w398, w396) -> (w397:errorcluster)
          }
        }
      }
      frame Error {
        n174 = control-ref of="This VI"() -> (w412:refnum<vi>)
        n175 = invoke class="VI" method="FP.Close"(reference=w412) -> ()  [unwired: 2 in, 3 out]
      }
    }
  }
  "error out" <- w9
  "RF Powers out" <- w1
  "Canceled" <- w8
  "Parameters" <- w10
